vi "Handle Errors.vi"(8 "error in":errorcluster, 11 "PAS in":refnum<class "PAS.lvclass">) -> (0 "error out":errorcluster, 2 "errors":errorcluster[](array[cluster]), 3 "PAS out":refnum<class "PAS.lvclass">)   [LabVIEW 2014, in "PAS.lvclass"]
doc: "Handle errors thrown by the data acquisition system. Most can be thrown out with no deleterious effect on performance - simply report them via whatever means provided by the current instance of the PAS class. If a data acquisition error is thrown however, make sure that the tasks associated with these are restarted to avoid more errors down the line."
uses:
  PAS.lvclass
  Instrument/Instrument.lvclass
  Instrument/state.ctl
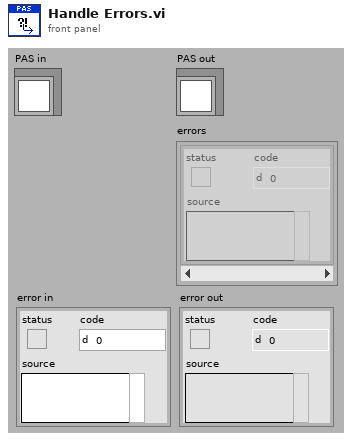
[diagram p1: front panel]
types:
  T1 = typedef "Instrument.lvclass/state.ctl" = enum8{"Configure", "Acquire", "Wait", "Quit", "Handle Error", "NOOP"}
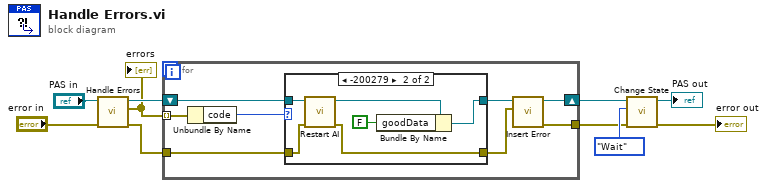
[diagram p0: block diagram]
diagram:
  n1 = call-parent "Handle Errors.vi"("error in"="error in", "Instrument in"="PAS in") -> ("error out"=w7:errorcluster, "errors"=w6:errorcluster[], "Instrument out"=w8:refnum<class "PAS.lvclass">)  [unwired: 7 in]
  "errors" <- w6
  n2 = for {
    tunnel: w6 -> [w12] mode=indexing
    shift-right: [w14] -> w4
    shift-left: w8 -> [w17]
    tunnel: w7 -> [w11]
    tunnel: [w13] -> w2
    n3 = Unbundle By Name(w12) -> ("code"=w18:i32)
    n4 = case shown="-200279" w18 {
      tunnel: w17 -> [w20 w26]
      tunnel: [w20 w22] -> w16
      tunnel: w11 -> [w19 w25]
      tunnel: [w19 w24] -> w15
      frame 0, Default {
      }
      frame -200279 {
        n5 = call "Restart AI.vi"("error in"=w25, "PAS in"=w26) -> ("error out"=w24:errorcluster, "PAS out"=w23:refnum<class "PAS.lvclass">)  [unwired: 8 in]
        n6 = Bundle By Name(cluster=w23, "goodData"=FALSE) -> (w22:refnum<class "PAS.lvclass">)
      }
    }
    n7 = call "Insert Error.vi"("err"=w15, "Instrument in"=w16) -> ("error out"=w13:errorcluster, "Instrument out"=w14:refnum<class "PAS.lvclass">)  [unwired: 7 in, 1 out]
  }
  n8 = call "Change State.vi"("error in"=w2, "instr state"=state."Wait", "Instrument in"=w4) -> ("error out"=→"error out":errorcluster, "Instrument out"=→"PAS out":refnum<class "PAS.lvclass">)  [unwired: 7 in]
